vi "Read Laundry.vi"(8 "error in (no error)":errorcluster, 11 "Housekeeping in":refnum<class "Housekeeping.lvclass">) -> (0 "error out":errorcluster, 2 "Laundry":bool, 3 "Housekeeping out":refnum<class "Housekeeping.lvclass">)   [LabVIEW 2023, in "Room Service Types.lvlib" / "Housekeeping.lvclass"]
uses:
  Housekeeping.lvclass
  Housekeeping.lvclass/Housekeeping.ctl
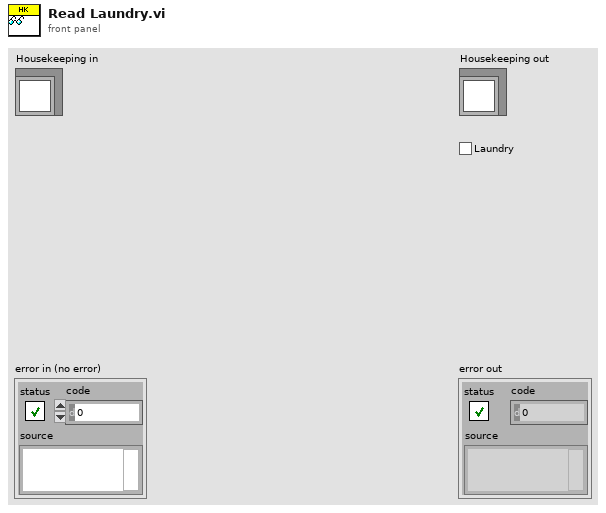
[diagram p1: front panel]
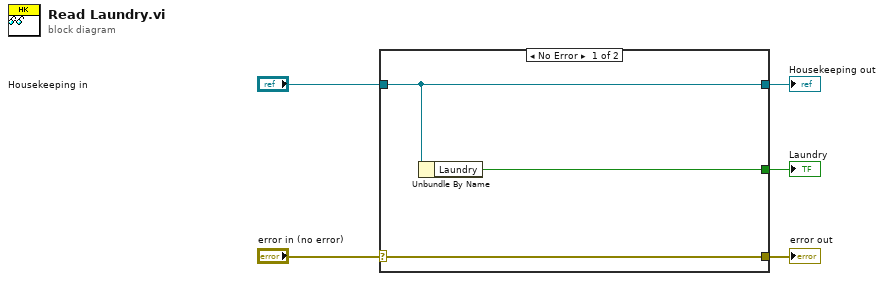
[diagram p0: block diagram]
diagram:
  n1 = case shown="No Error" "error in (no error)" {
    selector: "error in (no error)" -> [w8 w9]
    tunnel: [w8 w9] -> w4
    tunnel: [w7 w10] -> w2
    tunnel: "Housekeeping in" -> [w7 w10]
    tunnel: [w6 _] -> w1
    frame No Error {
      n2 = Unbundle By Name(w7) -> ("Laundry"=w6:bool)
    }
    frame Error {
    }
  }
  "error out" <- w4
  "Housekeeping out" <- w2
  "Laundry" <- w1
